vi "RI_OPEN_JT.vi"(2 "error in (no error)":errorcluster) -> (0 "error out":errorcluster, 1 "connection ID":refnum<k5>)   [LabVIEW 2019]
uses:
  Instrument_Setup.vi
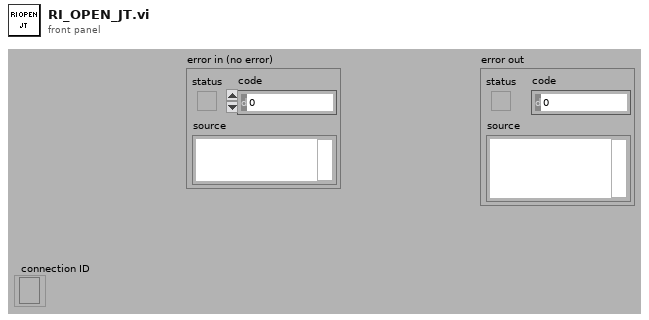
[diagram p1: front panel]
types:
  T1 = cluster{"Mode":enum16{"Standard", "Buffered", "CRLF", "Immediate"}, "Bytes to Read":i32, "IP Address":string, "Remote Port":i32, "Timeout":i32}
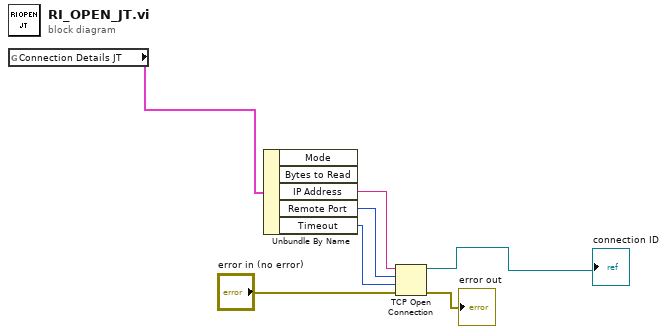
[diagram p0: block diagram]
diagram:
  n1 = global read "Instrument_Setup.vi" "Connection Details JT"() -> (w1:T1)
  n2 = Unbundle By Name(w1) -> ("IP Address"=w5:string, "Remote Port"=w4:i32, "Timeout"=w3:i32)  [unwired: 2 out]
  n3 = TCP Open Connection(address=w5, remote port or service name=w4, timeout ms (60000)=w3, error in (no error)="error in (no error)") -> (connection ID=→"connection ID":refnum<k5>, error out=→"error out":errorcluster)  [unwired: 1 in]
